vi "Begin.vi"(11 "Image Size":T1=enum."160x120") -> (0 "error out":errorcluster)   [LabVIEW 2011]
doc: "Called before other user functions, this VI is expected to open initial I/O refnums, load in file data, and do all program initialization. Notice that the <B>error out</B> terminal is simply used for data flow. Wiring it to other structures or subVIs ensures that this VI runs first."
uses:
  <vilib>/Rock Robotics/WPI/Camera/WPI_CameraImageSize.ctl
  <vilib>/Rock Robotics/SystemInterfaces/DIO/FPGA_DIOPWMChannel.ctl
  <vilib>/Rock Robotics/WPI/Joystick/WPI_JoystickDeviceEnum.ctl
  <vilib>/Rock Robotics/WPI/Camera/WPI_CameraWhite Balance Values.ctl
  <vilib>/Rock Robotics/WPI/Camera/WPI_CameraExposure Values.ctl
  <vilib>/Rock Robotics/WPI/Camera/WPI_CameraFrameRate.ctl
  <vilib>/Rock Robotics/SystemInterfaces/DIO/FPGA_DIOChannel.ctl
  <vilib>/Rock Robotics/SystemInterfaces/Typedef/FPGA_TypedefDigitalModule.ctl
  <vilib>/Rock Robotics/SystemInterfaces/Typedef/FPGA_TypedefSolenoidModule.ctl
  <vilib>/Rock Robotics/WPI/Solenoid/WPI_SolenoidChannel.ctl
  <vilib>/Rock Robotics/WPI/Encoder/WPI_EncoderType.ctl
  <vilib>/Rock Robotics/SystemInterfaces/DIO/FPGA_DIORelayChannel.ctl
  <vilib>/Rock Robotics/SystemInterfaces/AI/FPGA_AIGyroChannel.ctl
  <vilib>/Rock Robotics/SystemInterfaces/Typedef/FPGA_TypedefAnalogModuleForGyro.ctl
  <vilib>/Rock Robotics/WPI/Solenoid/WPI_SolenoidOpenSingle.vi
  <vilib>/Rock Robotics/WPI/Counter/WPI_CounterDigitalInputToDigitalSource.vi
  <vilib>/Rock Robotics/WPI/RobotDrive/WPI_RobotDriveOpen2MotorWithJaguar.vi
  <vilib>/Rock Robotics/WPI/RobotDrive/WPI_RobotDriveOpen4MotorWithJaguar.vi
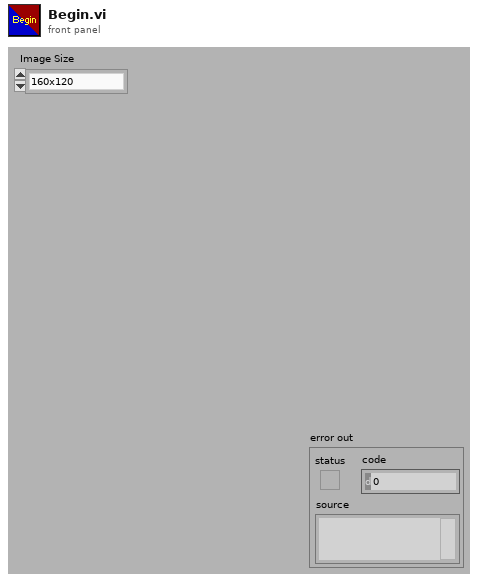
[diagram p1: front panel]
types:
  T1 = typedef "WPI_CameraImageSize.ctl" = enum16{"640x480", "320x240", "160x120"}
  T2 = typedef "FPGA_DIOChannel.ctl" = enum8{"DIO 1", "DIO 2", "DIO 3", "DIO 4", "DIO 5", "DIO 6", "DIO 7", "DIO 8", "DIO 9", "DIO 10", "DIO 11", "DIO 12", "DIO 13", "DIO 14", "Invalid"}
  T3 = typedef "FPGA_TypedefDigitalModule.ctl" = enum16{"Digital Module 1", "Digital Module 2"}
  T4 = typedef "WPI_EncoderType.ctl" = enum16{"1x", "2x", "4x"}
  T5 = typedef "FPGA_TypedefSolenoidModule.ctl" = enum16{"Solenoid Module 1", "Solenoid Module 2"}
  T6 = typedef "WPI_SolenoidChannel.ctl" = enum8{"Solenoid 1", "Solenoid 2", "Solenoid 3", "Solenoid 4", "Solenoid 5", "Solenoid 6", "Solenoid 7", "Solenoid 8", "Invalid"}
  T7 = typedef "FPGA_TypedefAnalogModuleForGyro.ctl" = enum16{"Analog Module 1"}
  T8 = typedef "FPGA_AIGyroChannel.ctl" = enum8{"AI 1", "AI 2", "Invalid"}
  T9 = typedef "FPGA_DIORelayChannel.ctl" = enum8{"Relay 1", "Relay 2", "Relay 3", "Relay 4", "Relay 5", "Relay 6", "Relay 7", "Relay 8", "Invalid"}
  T10 = typedef "FPGA_DIOPWMChannel.ctl" = enum8{"PWM 1", "PWM 2", "PWM 3", "PWM 4", "PWM 5", "PWM 6", "PWM 7", "PWM 8", "PWM 9", "PWM 10", "Invalid"}
  T11 = typedef "WPI_JoystickDeviceEnum.ctl" = enum16{"USB 1", "USB 2", "USB 3", "USB 4", "Kinect 1", "Kinect 2"}
  T12 = typedef "WPI_CameraFrameRate.ctl" = u32
  T13 = typedef "WPI_CameraExposure Values.ctl" = enum16{"Auto", "Flicker-free 50 Hz", "Flicker-free 60 Hz", "Hold current"}
  T14 = typedef "WPI_CameraWhite Balance Values.ctl" = enum16{"Auto", "Fixed indoor", "Fixed outdoor 1", "Fixed outdoor 2", "Fixed fluorescent 1", "Fixed fluorescent 2", "Hold current"}
  T15 = typedef "WPI_CompressorDevRef.ctl" = cluster{"DevStatus":errorcluster, "TaskVI":refnum<vi>, "Enabled":bool, "FIFO_enabled":refnum<k33>, "FIFO_relay":refnum<k33>}
  T16 = typedef "WPI_SolenoidDevRef.ctl" = cluster{"DevStatus":errorcluster, "Solenoid Module":T5, "Forward Solenoid Channel":T6, "Reverse Solenoid Channel":T6}
  T17 = typedef "WPI_DigitalInputDevRef.ctl" = cluster{"DevStatus":errorcluster, "DIO Channel":T2, "Digital Module":T3}
  T18 = typedef "WPI_JoystickDevRef.ctl" = cluster{"Device":T11}
  T19 = typedef "WPI_CameraDevRef.ctl" = cluster{"Camera Address":string, "CameraStatus":errorcluster, "Session ID":T20}
  T20 = typedef "WPI_CameraSessionID.ctl" = i32
  T21 = typedef "WPI_ServoDeviceRef.ctl" = cluster{"DeviceStatus":errorcluster, "Digital Module":T3, "PWM Channel":T10, "DeadBand":T22}
  T22 = typedef "WPI_PWMDeadband.ctl" = cluster{"Name":string, "maxPositivePwm":i32, "minPositivePwm":i32, "centerPwm":i32, "maxNegativePwm":i32, "minNegativePwm":i32, "angularRange":u16}
  T23 = typedef "WPI_RobotDriveDevRef.ctl" = cluster{"DevStatus":errorcluster, "Motors[]":T24[], "Square Inputs":bool, "Max Output":dbl}
  T24 = typedef "WPI_MotorControlDeviceRef.ctl" = cluster{"DeviceStatus":errorcluster, "Type":enum16{"PWM", "CAN"}, "PWM":cluster{"Digital Module":T3, "PWM Channel":T10, "DeadBand":T22}, "CAN":cluster{"Device Number":u8, "Control Mode":T25, "Semaphore":T26, "Max Vout":dbl}, "Invert":bool, "TransformRef":T27, "InvTransformRef":T27}
  T25 = typedef "WPI_CANJaguar_ControlMode.ctl" = enum8{"Percent VBus", "Current", "Speed", "Position", "Voltage"}
  T26 = typedef "Semaphore RefNum" = refnum<k1>
  T27 = typedef "WPI_PWMTransform_ConPane.ctl" = refnum<vi>
  T28 = typedef "FPGA_CounterEncoderSourceConvertionLVSourceType.ctl" = cluster{"DevStatus":errorcluster, "AnalogTriggerMode?":bool, "DigitalMode":cluster{"Digital Module":T3, "DIO Channel":T29}, "AnalogTriggerMode":cluster{"AnalogTriggerIndex":T30, "OutputType":T31}}
  T29 = typedef "FPGA_DIODigitalSourceChannel.ctl" = enum8{"DIO 1", "DIO 2", "DIO 3", "DIO 4", "DIO 5", "DIO 6", "DIO 7", "DIO 8", "DIO 9", "DIO 10", "DIO 11", "DIO 12", "DIO 13", "DIO 14", "Disabled"}
  T30 = typedef "FPGA_AnalogTriggerIndex.ctl" = enum8{"Trig 0", "Trig 1", "Trig 2", "Trig 3", "Trig 4", "Trig 5", "Trig 6", "Trig 7", "Invalid"}
  T31 = typedef "FPGA_AnalogTriggerOutType.ctl" = enum16{"InWindow", "TriggerState", "Rising", "Falling"}
  T32 = typedef "WPI_EncoderDevRef.ctl" = cluster{"DevStatus":errorcluster, "EncoderIndex":T33, "CounterIndex":T34, "DistancePerCount":dbl, "Decoding Type":T4}
  T33 = typedef "FPGA_EncoderIdx.ctl" = enum8{"Enc 0", "Enc 1", "Enc 2", "Enc 3", "Invalid"}
  T34 = typedef "FPGA_CounterCtrSystemIndex.ctl" = enum8{"Ctr 0", "Ctr 1", "Ctr 2", "Ctr 3", "Ctr 4", "Ctr 5", "Ctr 6", "Ctr 7", "Invalid"}
  T35 = typedef "WPI_GyroDevRef.ctl" = cluster{"DevStatus":errorcluster, "Analog Module":T36, "Analog Channel":T37, "Offset":dbl, "Gain (VoltsPerDegree/Second)":dbl}
  T36 = typedef "FPGA_TypedefAnalogModule.ctl" = enum16{"Analog Module 1", "Analog Module 2"}
  T37 = typedef "FPGA_AIChannel.ctl" = enum8{"AI 1", "AI 2", "AI 3", "AI 4", "AI 5", "AI 6", "AI 7", "AI 8", "Invalid"}
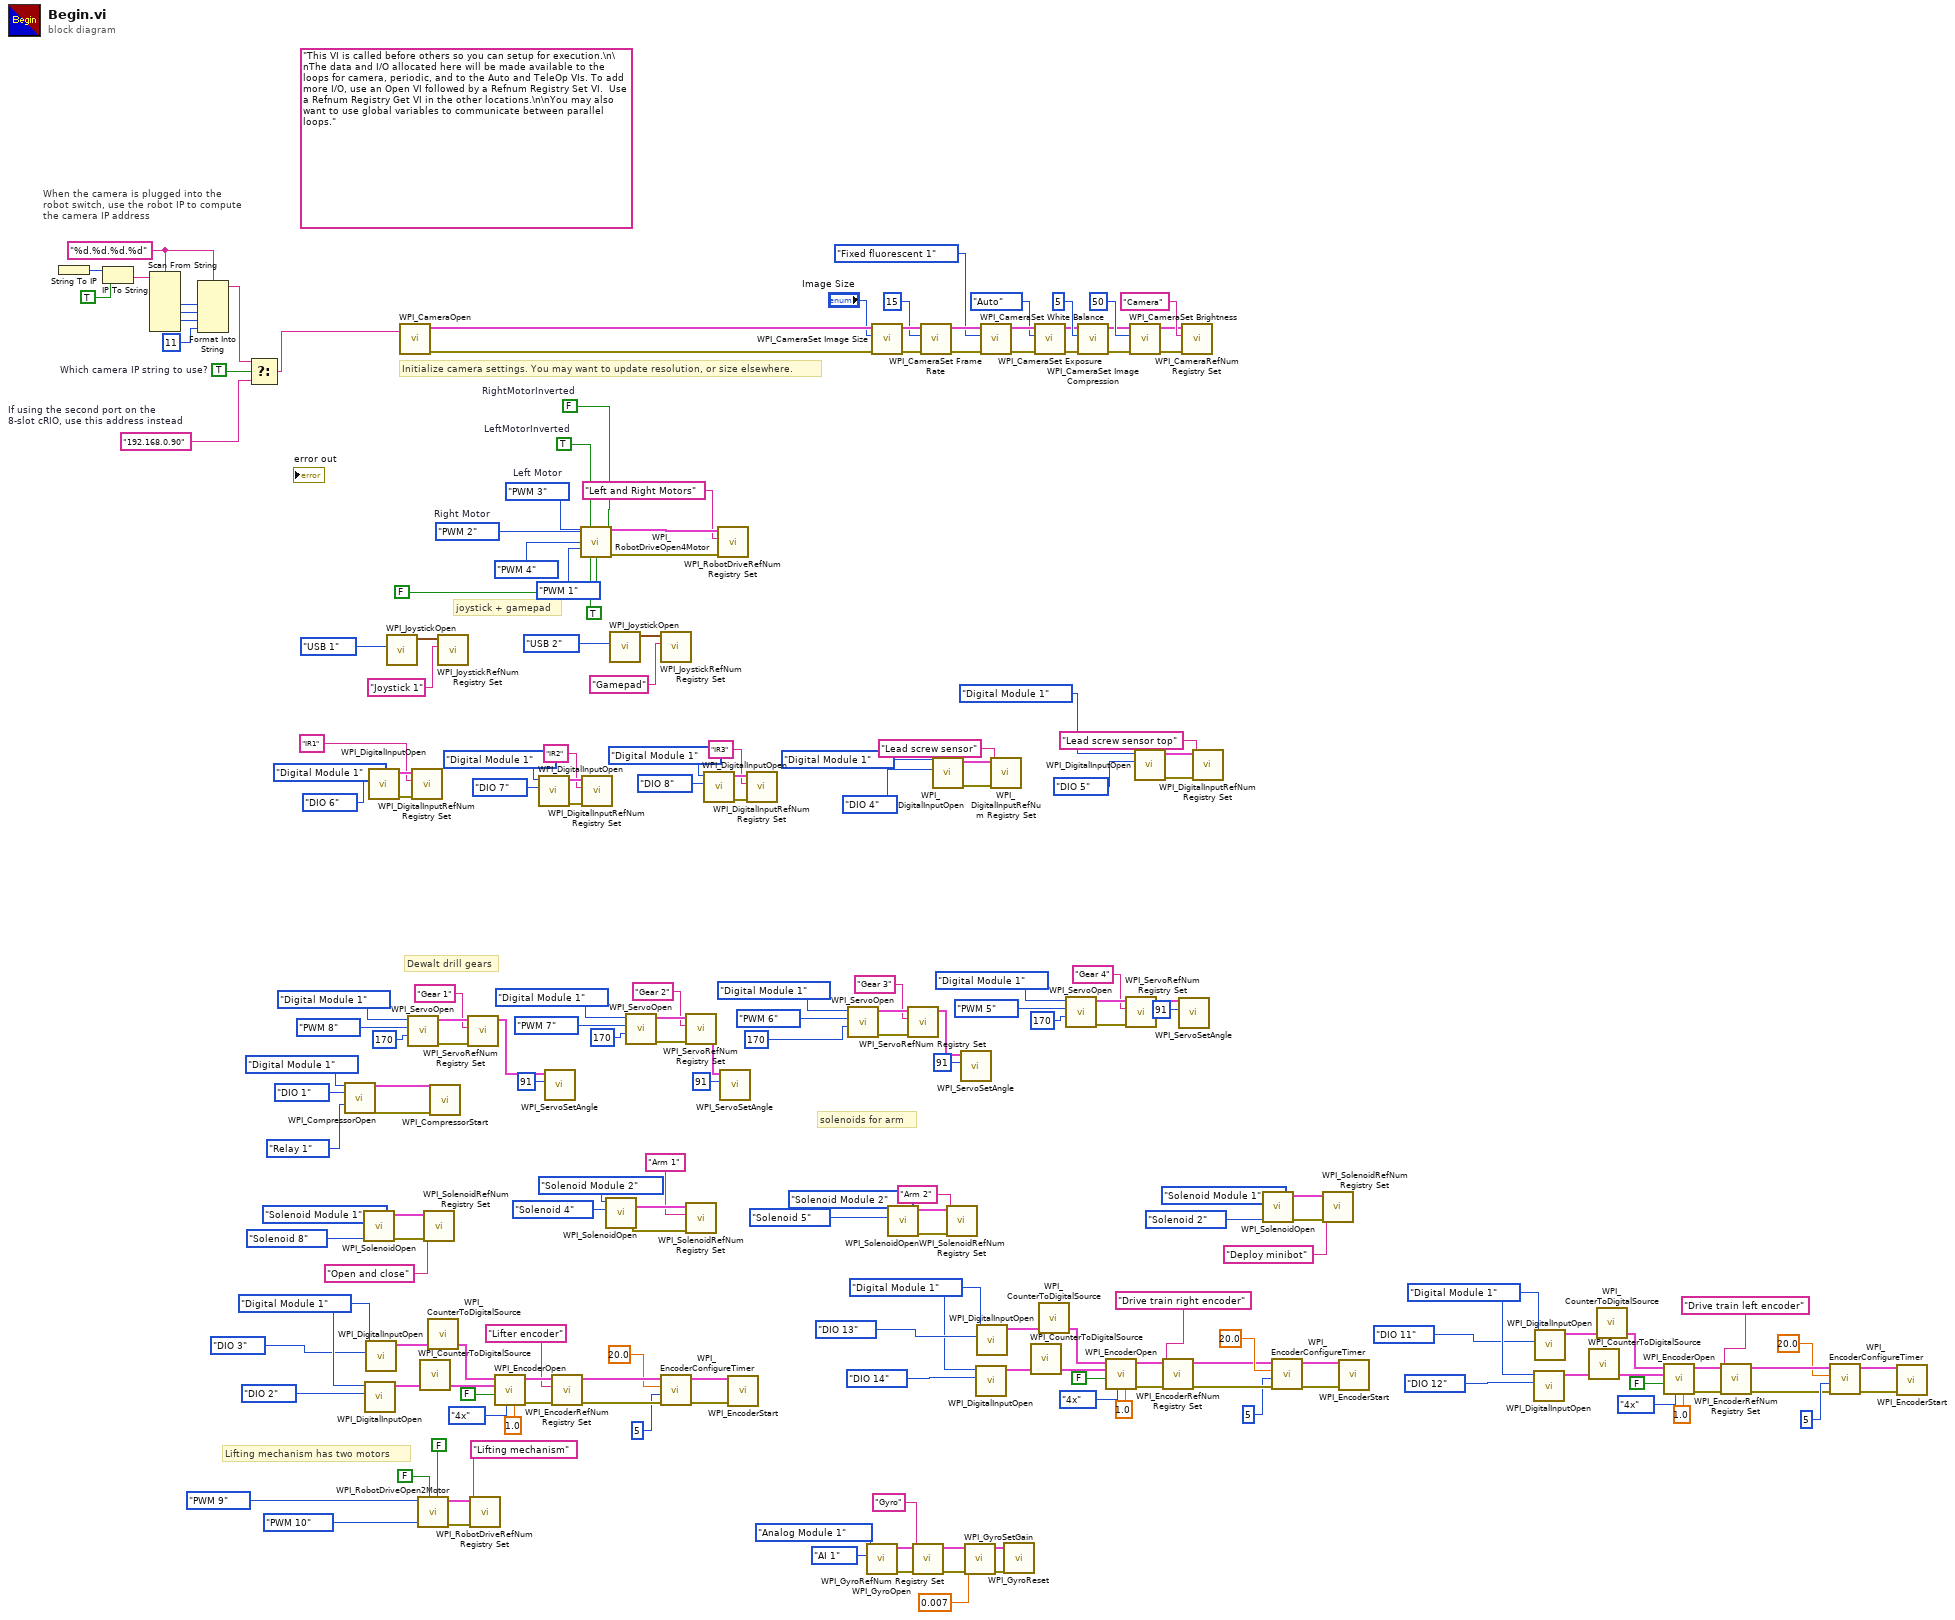
[diagram p0: block diagram]
diagram:
  w2 = TRUE  # Which camera IP string to use?
  w5 = "%d.%d.%d.%d" ("format string")
  w3 = "192.168.0.90"  # If using the second port on the 8-slot cRIO, use this address instead
  w33 = FPGA_TypedefDigitalModule."Digital Module 1" ("DIO Module (Slot 4)")
  w68 = FPGA_TypedefDigitalModule."Digital Module 1" ("DIO Module (Slot 4)")
  w106 = FPGA_TypedefDigitalModule."Digital Module 1" ("DIO Module (Slot 4)")
  (unwired) "This VI is called before others so you can setup for execution.\n\nThe data and I/O allocated here will be made available to the loops for camera, periodic, and to the Auto and TeleOp VIs. To add more I/O, use an Open VI followed by a Refnum Registry Set VI.  Use a Refnum Registry Get VI in the other locations.\n\nYou may also want to use global variables to communicate between parallel loops."
  w122 = FPGA_DIOPWMChannel."PWM 2"  # Right Motor
  w181 = FPGA_DIOPWMChannel."PWM 3"  # Left Motor
  w205 = TRUE  # LeftMotorInverted
  w206 = FALSE  # RightMotorInverted
  # "When the camera is plugged into the\nrobot switch, use the robot IP to compute\nthe camera IP address"
  # "Lifting mechanism has two motors"
  # "joystick + gamepad"
  # "Dewalt drill gears"
  # "solenoids for arm"
  # "Initialize camera settings. You may want to update resolution, or size elsewhere."
  n1 = String To IP() -> (0:w12:u32)  [unwired: 1 in]
  n2 = IP To String(1:TRUE ("dot notation? (F)"), 2:w12) -> (0:w10:string)
  n3 = Scan From String(format string=w5, input string=w10) -> (output 1=w9:i32, output 2=w8:i32, output 3=w7:i32)  [unwired: 7 in, 3 out]
  n4 = Format Into String(format string=w5, w9, w8, w7, 11 ("Compression")) -> (resulting string=w4:string)  [unwired: 2 in, 1 out]
  n5 = Select(t=w4, s=w2, f=w3) -> (s? t:f=w1:string)
  n6 = call <vilib>:"WPI_CompressorOpen.vi"("Pressure Switch Digital Module (Module 1)"=FPGA_TypedefDigitalModule."Digital Module 1" ("Pressure Switch DIO Module"), "Pressure Switch DIO Channel"=FPGA_DIOChannel."DIO 1", "Relay Channel"=FPGA_DIORelayChannel."Relay 1") -> ("CompressorDevRef"=w88:T15, "error out"=w87:errorcluster)  [unwired: 2 in, 9 out]
  n7 = call-poly <vilib>:"WPI_SolenoidOpen.vi"("Solenoid Channel"=WPI_SolenoidChannel."Solenoid 8", "Solenoid Module (Module 1)"=FPGA_TypedefSolenoidModule."Solenoid Module 1" ("Solenoid Module")) -> ("error out"=w133:errorcluster, "SolenoidDevRef"=w132:T16)  [unwired: 2 in, 6 out]
  n8 = call <vilib>:"WPI_DigitalInputOpen.vi"("DIO Channel"=FPGA_DIOChannel."DIO 2", "Digital Module (Module 1)"=w106) -> ("DigitalInputDevRef"=w108:T17)  [unwired: 1 in, 8 out]
  n9 = call <vilib>:"WPI_DigitalInputOpen.vi"("DIO Channel"=FPGA_DIOChannel."DIO 3", "Digital Module (Module 1)"=w106) -> ("DigitalInputDevRef"=w110:T17)  [unwired: 1 in, 8 out]
  n10 = call <vilib>:"WPI_DigitalInputOpen.vi"("DIO Channel"=FPGA_DIOChannel."DIO 6", "Digital Module (Module 1)"=FPGA_TypedefDigitalModule."Digital Module 1" ("DIO Module (Slot 4)")) -> ("error out"=w170:errorcluster, "DigitalInputDevRef"=w169:T17)  [unwired: 1 in, 7 out]
  n11 = call <vilib>:"WPI_JoystickOpen.vi"("JoystickDevice"=WPI_JoystickDeviceEnum."USB 1") -> ("JoystickDevRef"=w201:T18)  [unwired: 10 out]
  n12 = call <vilib>:"WPI_CameraOpen.vi"("Camera Address"=w1) -> ("error out"=w190:errorcluster, "CameraDevRef"=w191:T19)  [unwired: 1 in, 8 out]
  n13 = call <vilib>:"WPI_ServoOpen.vi"("Angular Range"=u16 170, "PWM Channel"=FPGA_DIOPWMChannel."PWM 8", "Digital Module (Module 1)"=FPGA_TypedefDigitalModule."Digital Module 1" ("DIO Module (Slot 4)")) -> ("error out"=w144:errorcluster, "ServoDeviceRef"=w145:T21)  [unwired: 1 in, 6 out]
  n14 = call <vilib>:"WPI_DigitalInputRefNum Registry Set.vi"("error in (no error)"=w170, "refnum name"="IR1", "DigitalInputDevRef"=w169) -> ()  [unwired: 9 out]
  n15 = call-poly <vilib>:"WPI_RobotDriveOpen2Motor.vi"("Right Motor Inverted"=FALSE, "Left Motor Inverted"=FALSE, "Right Motor"=FPGA_DIOPWMChannel."PWM 10" ("PWM Channel"), "Left Motor"=FPGA_DIOPWMChannel."PWM 9") -> ("error out"=w121:errorcluster, "RobotDriveDevRef"=w102:T23)  [unwired: 1 in, 5 out]
  n16 = call-poly <vilib>:"WPI_CounterToDigitalSource.vi"("DigitalInputDevRef"=w108) -> ("Digital Source"=w107:T28)  [unwired: 6 out]
  n17 = call <vilib>:"WPI_SolenoidRefNum Registry Set.vi"("error in (no error)"=w133, "refnum name"="Open and close", "SolenoidDevRef"=w132) -> ()  [unwired: 9 out]
  n18 = call-poly <vilib>:"WPI_CounterToDigitalSource.vi"("DigitalInputDevRef"=w110) -> ("Digital Source"=w109:T28)  [unwired: 6 out]
  n19 = call <vilib>:"WPI_CompressorStart.vi"("error in (no error)"=w87, "CompressorDevRef"=w88) -> ()  [unwired: 10 out]
  n20 = call <vilib>:"WPI_JoystickRefNum Registry Set.vi"("refnum name"="Joystick 1", "JoystickDevRef"=w201) -> ()  [unwired: 1 in, 9 out]
  n21 = call <vilib>:"WPI_ServoRefNum Registry Set.vi"("error in (no error)"=w144, "refnum name"="Gear 1", "ServoDeviceRef"=w145) -> ("ServoDeviceRef"=w20:T21)  [unwired: 8 out]
  n22 = call <vilib>:"WPI_RobotDriveRefNum Registry Set.vi"("error in (no error)"=w121, "refnum name"="Lifting mechanism", "RobotDriveDevRef"=w102) -> ()  [unwired: 9 out]
  n23 = call <vilib>:"WPI_EncoderOpen.vi"("DistancePerCount"=1.0, "Decoding Type"=WPI_EncoderType."4x", "Invert Direction (False)"=FALSE, "BSource"=w107, "ASource"=w109) -> ("error out"=w118:errorcluster, "EncoderDevRef"=w117:T32)  [unwired: 3 in, 2 out]
  n24 = call <vilib>:"WPI_DigitalInputOpen.vi"("DIO Channel"=FPGA_DIOChannel."DIO 7", "Digital Module (Module 1)"=FPGA_TypedefDigitalModule."Digital Module 1" ("DIO Module (Slot 4)")) -> ("error out"=w168:errorcluster, "DigitalInputDevRef"=w167:T17)  [unwired: 1 in, 7 out]
  n25 = call <vilib>:"WPI_ServoSetAngle.vi"("Angle"=91, "ServoDeviceRef"=w20) -> ()  [unwired: 1 in, 9 out]
  n26 = call <vilib>:"WPI_EncoderRefNum Registry Set.vi"("error in (no error)"=w118, "refnum name"="Lifter encoder", "EncoderDevRef"=w117) -> ("error out"=w83:errorcluster, "EncoderDevRef"=w84:T32)  [unwired: 7 out]
  n27 = call-poly <vilib>:"WPI_RobotDriveOpen4Motor.vi"("Rear Left Motor"=w181, "Rear Left Motor Inverted"=w205, "Rear Right Motor Inverted"=w206, "Rear Right Motor"=w122, "Front Left Motor"=FPGA_DIOPWMChannel."PWM 4", "Front Right Motor"=FPGA_DIOPWMChannel."PWM 1", "Front Left Motor Inverted"=TRUE, "Front Right Motor Inverted"=FALSE) -> ("RobotDriveDevRef"=w203:T23, "error out"=w199:errorcluster)  [unwired: 1 in, 5 out]
  n28 = call <vilib>:"WPI_DigitalInputRefNum Registry Set.vi"("error in (no error)"=w168, "refnum name"="IR2", "DigitalInputDevRef"=w167) -> ()  [unwired: 9 out]
  n29 = call-poly <vilib>:"WPI_SolenoidOpen.vi"("Solenoid Channel"=WPI_SolenoidChannel."Solenoid 4", "Solenoid Module (Module 1)"=FPGA_TypedefSolenoidModule."Solenoid Module 2" ("Solenoid Module")) -> ("error out"=w131:errorcluster, "SolenoidDevRef"=w130:T16)  [unwired: 2 in, 6 out]
  n30 = call <vilib>:"WPI_JoystickOpen.vi"("JoystickDevice"=WPI_JoystickDeviceEnum."USB 2") -> ("JoystickDevRef"=w124:T18)  [unwired: 10 out]
  n31 = call <vilib>:"WPI_ServoOpen.vi"("Angular Range"=u16 170, "PWM Channel"=FPGA_DIOPWMChannel."PWM 7", "Digital Module (Module 1)"=FPGA_TypedefDigitalModule."Digital Module 1" ("DIO Module (Slot 4)")) -> ("error out"=w146:errorcluster, "ServoDeviceRef"=w149:T21)  [unwired: 1 in, 6 out]
  n32 = call <vilib>:"WPI_JoystickRefNum Registry Set.vi"("refnum name"="Gamepad", "JoystickDevRef"=w124) -> ()  [unwired: 1 in, 9 out]
  n33 = call <vilib>:"WPI_EncoderConfigureTimer.vi"("error in (no error)"=w83, "Number Samples to Average"=u8 5, "Minimum Rate"=20.0, "EncoderDevRef"=w84) -> ("error out"=w79:errorcluster, "EncoderDevRef"=w80:T32)  [unwired: 6 out]
  n34 = call <vilib>:"WPI_ServoRefNum Registry Set.vi"("error in (no error)"=w146, "refnum name"="Gear 2", "ServoDeviceRef"=w149) -> ("ServoDeviceRef"=w18:T21)  [unwired: 8 out]
  n35 = call <vilib>:"WPI_SolenoidRefNum Registry Set.vi"("error in (no error)"=w131, "refnum name"="Arm 1", "SolenoidDevRef"=w130) -> ()  [unwired: 9 out]
  n36 = call <vilib>:"WPI_DigitalInputOpen.vi"("DIO Channel"=FPGA_DIOChannel."DIO 8", "Digital Module (Module 1)"=FPGA_TypedefDigitalModule."Digital Module 1" ("DIO Module (Slot 4)")) -> ("error out"=w166:errorcluster, "DigitalInputDevRef"=w165:T17)  [unwired: 1 in, 7 out]
  n37 = call <vilib>:"WPI_RobotDriveRefNum Registry Set.vi"("error in (no error)"=w199, "refnum name"="Left and Right Motors", "RobotDriveDevRef"=w203) -> ()  [unwired: 9 out]
  n38 = call <vilib>:"WPI_ServoSetAngle.vi"("Angle"=91, "ServoDeviceRef"=w18) -> ()  [unwired: 1 in, 9 out]
  n39 = call <vilib>:"WPI_EncoderStart.vi"("error in (no error)"=w79, "EncoderDevRef"=w80) -> ()  [unwired: 10 out]
  n40 = call <vilib>:"WPI_DigitalInputRefNum Registry Set.vi"("error in (no error)"=w166, "refnum name"="IR3", "DigitalInputDevRef"=w165) -> ()  [unwired: 9 out]
  n41 = call <vilib>:"WPI_ServoOpen.vi"("Angular Range"=u16 170, "PWM Channel"=FPGA_DIOPWMChannel."PWM 6", "Digital Module (Module 1)"=FPGA_TypedefDigitalModule."Digital Module 1" ("DIO Module (Slot 4)")) -> ("error out"=w148:errorcluster, "ServoDeviceRef"=w147:T21)  [unwired: 1 in, 6 out]
  n42 = call <vilib>:"WPI_GyroOpen.vi"("Analog Channel"=FPGA_AIGyroChannel."AI 1", "Analog Module (Module 1)"=FPGA_TypedefAnalogModuleForGyro."Analog Module 1" ("Analog Module (Slot 1)")) -> ("error out"=w57:errorcluster, "GyroDevRef"=w56:T35)  [unwired: 4 in, 4 out]
  n43 = call <vilib>:"WPI_CameraSet Image Size.vi"("error in (no error)"=w190, "Image Size"="Image Size", "CameraDevRef"=w191) -> ("error out"=w189:errorcluster, "CameraDevRef Out"=w192:T19)  [unwired: 7 out]
  n44 = call-poly <vilib>:"WPI_SolenoidOpen.vi"("Solenoid Channel"=WPI_SolenoidChannel."Solenoid 5", "Solenoid Module (Module 1)"=FPGA_TypedefSolenoidModule."Solenoid Module 2" ("Solenoid Module")) -> ("error out"=w47:errorcluster, "SolenoidDevRef"=w46:T16)  [unwired: 2 in, 6 out]
  n45 = call <vilib>:"WPI_ServoRefNum Registry Set.vi"("error in (no error)"=w148, "refnum name"="Gear 3", "ServoDeviceRef"=w147) -> ("ServoDeviceRef"=w16:T21)  [unwired: 8 out]
  n46 = call <vilib>:"WPI_GyroRefNum Registry Set.vi"("error in (no error)"=w57, "refnum name"="Gyro", "GyroDevRef"=w56) -> ("error out"=w44:errorcluster, "GyroDevRef"=w43:T35)  [unwired: 7 out]
  n47 = call <vilib>:"WPI_CameraSet Frame Rate.vi"("error in (no error)"=w189, "Frame Rate (fps)"=T12 15, "CameraDevRef"=w192) -> ("error out"=w188:errorcluster, "CameraDevRef Out"=w194:T19)  [unwired: 7 out]
  n48 = call <vilib>:"WPI_DigitalInputOpen.vi"("DIO Channel"=FPGA_DIOChannel."DIO 4", "Digital Module (Module 1)"=FPGA_TypedefDigitalModule."Digital Module 1" ("DIO Module (Slot 4)")) -> ("error out"=w115:errorcluster, "DigitalInputDevRef"=w114:T17)  [unwired: 1 in, 7 out]
  n49 = call <vilib>:"WPI_SolenoidRefNum Registry Set.vi"("error in (no error)"=w47, "refnum name"="Arm 2", "SolenoidDevRef"=w46) -> ()  [unwired: 9 out]
  n50 = call <vilib>:"WPI_ServoSetAngle.vi"("Angle"=91, "ServoDeviceRef"=w16) -> ()  [unwired: 1 in, 9 out]
  n51 = call <vilib>:"WPI_GyroSetGain.vi"("error in (no error)"=w44, "Gain (VoltsPerDegree/Second)"=0.007, "GyroDevRef"=w43) -> ("error out"=w22:errorcluster, "GyroDevRef"=w21:T35)  [unwired: 7 out]
  n52 = call <vilib>:"WPI_DigitalInputOpen.vi"("DIO Channel"=FPGA_DIOChannel."DIO 14", "Digital Module (Module 1)"=w68) -> ("DigitalInputDevRef"=w66:T17)  [unwired: 1 in, 8 out]
  n53 = call <vilib>:"WPI_DigitalInputOpen.vi"("DIO Channel"=FPGA_DIOChannel."DIO 13", "Digital Module (Module 1)"=w68) -> ("DigitalInputDevRef"=w64:T17)  [unwired: 1 in, 8 out]
  n54 = call <vilib>:"WPI_CameraSet White Balance.vi"("error in (no error)"=w188, "White Balance"=WPI_CameraWhite_Balance_Values."Fixed fluorescent 1", "CameraDevRef"=w194) -> ("error out"=w187:errorcluster, "CameraDevRef Out"=w193:T19)  [unwired: 7 out]
  n55 = call <vilib>:"WPI_DigitalInputRefNum Registry Set.vi"("error in (no error)"=w115, "refnum name"="Lead screw sensor", "DigitalInputDevRef"=w114) -> ()  [unwired: 9 out]
  n56 = call <vilib>:"WPI_GyroReset.vi"("error in (no error)"=w22, "GyroDevRef"=w21) -> ()  [unwired: 10 out]
  n57 = call-poly <vilib>:"WPI_CounterToDigitalSource.vi"("DigitalInputDevRef"=w66) -> ("Digital Source"=w67:T28)  [unwired: 6 out]
  n58 = call <vilib>:"WPI_CameraSet Exposure.vi"("error in (no error)"=w187, "Exposure"=WPI_CameraExposure_Values."Auto", "CameraDevRef"=w193) -> ("error out"=w186:errorcluster, "CameraDevRef Out"=w196:T19)  [unwired: 7 out]
  n59 = call-poly <vilib>:"WPI_CounterToDigitalSource.vi"("DigitalInputDevRef"=w64) -> ("Digital Source"=w65:T28)  [unwired: 6 out]
  n60 = call <vilib>:"WPI_ServoOpen.vi"("Angular Range"=u16 170, "PWM Channel"=FPGA_DIOPWMChannel."PWM 5", "Digital Module (Module 1)"=FPGA_TypedefDigitalModule."Digital Module 1" ("DIO Module (Slot 4)")) -> ("error out"=w143:errorcluster, "ServoDeviceRef"=w142:T21)  [unwired: 1 in, 6 out]
  n61 = call <vilib>:"WPI_CameraSet Image Compression.vi"("error in (no error)"=w186, "Compression"=5, "CameraDevRef"=w196) -> ("error out"=w185:errorcluster, "CameraDevRef Out"=w195:T19)  [unwired: 7 out]
  n62 = call <vilib>:"WPI_EncoderOpen.vi"("DistancePerCount"=1.0, "Decoding Type"=WPI_EncoderType."4x", "Invert Direction (False)"=FALSE, "BSource"=w67, "ASource"=w65) -> ("error out"=w61:errorcluster, "EncoderDevRef"=w62:T32)  [unwired: 3 in, 2 out]
  n63 = call <vilib>:"WPI_ServoRefNum Registry Set.vi"("error in (no error)"=w143, "refnum name"="Gear 4", "ServoDeviceRef"=w142) -> ("ServoDeviceRef"=w14:T21)  [unwired: 8 out]
  n64 = call <vilib>:"WPI_CameraSet Brightness.vi"("error in (no error)"=w185, "Brightness"=50, "CameraDevRef"=w195) -> ("error out"=w183:errorcluster, "CameraDevRef Out"=w184:T19)  [unwired: 7 out]
  n65 = call <vilib>:"WPI_DigitalInputOpen.vi"("DIO Channel"=FPGA_DIOChannel."DIO 5", "Digital Module (Module 1)"=FPGA_TypedefDigitalModule."Digital Module 1" ("DIO Module (Slot 4)")) -> ("error out"=w94:errorcluster, "DigitalInputDevRef"=w95:T17)  [unwired: 1 in, 7 out]
  n66 = call <vilib>:"WPI_EncoderRefNum Registry Set.vi"("error in (no error)"=w61, "refnum name"="Drive train right encoder", "EncoderDevRef"=w62) -> ("error out"=w75:errorcluster, "EncoderDevRef"=w74:T32)  [unwired: 7 out]
  n67 = call <vilib>:"WPI_ServoSetAngle.vi"("Angle"=91, "ServoDeviceRef"=w14) -> ()  [unwired: 1 in, 9 out]
  n68 = call <vilib>:"WPI_CameraRefNum Registry Set.vi"("error in (no error)"=w183, "refnum name"="Camera", "CameraDevRef"=w184) -> ()  [unwired: 9 out]
  n69 = call <vilib>:"WPI_DigitalInputRefNum Registry Set.vi"("error in (no error)"=w94, "refnum name"="Lead screw sensor top", "DigitalInputDevRef"=w95) -> ()  [unwired: 9 out]
  n70 = call-poly <vilib>:"WPI_SolenoidOpen.vi"("Solenoid Channel"=WPI_SolenoidChannel."Solenoid 2", "Solenoid Module (Module 1)"=FPGA_TypedefSolenoidModule."Solenoid Module 1" ("Solenoid Module")) -> ("error out"=w52:errorcluster, "SolenoidDevRef"=w53:T16)  [unwired: 2 in, 6 out]
  n71 = call <vilib>:"WPI_EncoderConfigureTimer.vi"("error in (no error)"=w75, "Number Samples to Average"=u8 5, "Minimum Rate"=20.0, "EncoderDevRef"=w74) -> ("error out"=w78:errorcluster, "EncoderDevRef"=w77:T32)  [unwired: 6 out]
  n72 = call <vilib>:"WPI_SolenoidRefNum Registry Set.vi"("error in (no error)"=w52, "refnum name"="Deploy minibot", "SolenoidDevRef"=w53) -> ()  [unwired: 9 out]
  n73 = call <vilib>:"WPI_EncoderStart.vi"("error in (no error)"=w78, "EncoderDevRef"=w77) -> ()  [unwired: 10 out]
  n74 = call <vilib>:"WPI_DigitalInputOpen.vi"("DIO Channel"=FPGA_DIOChannel."DIO 12", "Digital Module (Module 1)"=w33) -> ("DigitalInputDevRef"=w35:T17)  [unwired: 1 in, 8 out]
  n75 = call <vilib>:"WPI_DigitalInputOpen.vi"("DIO Channel"=FPGA_DIOChannel."DIO 11", "Digital Module (Module 1)"=w33) -> ("DigitalInputDevRef"=w37:T17)  [unwired: 1 in, 8 out]
  n76 = call-poly <vilib>:"WPI_CounterToDigitalSource.vi"("DigitalInputDevRef"=w35) -> ("Digital Source"=w34:T28)  [unwired: 6 out]
  n77 = call-poly <vilib>:"WPI_CounterToDigitalSource.vi"("DigitalInputDevRef"=w37) -> ("Digital Source"=w36:T28)  [unwired: 6 out]
  n78 = call <vilib>:"WPI_EncoderOpen.vi"("DistancePerCount"=1.0, "Decoding Type"=WPI_EncoderType."4x", "Invert Direction (False)"=FALSE, "BSource"=w34, "ASource"=w36) -> ("error out"=w40:errorcluster, "EncoderDevRef"=w39:T32)  [unwired: 3 in, 2 out]
  n79 = call <vilib>:"WPI_EncoderRefNum Registry Set.vi"("error in (no error)"=w40, "refnum name"="Drive train left encoder", "EncoderDevRef"=w39) -> ("error out"=w26:errorcluster, "EncoderDevRef"=w27:T32)  [unwired: 7 out]
  n80 = call <vilib>:"WPI_EncoderConfigureTimer.vi"("error in (no error)"=w26, "Number Samples to Average"=u8 5, "Minimum Rate"=20.0, "EncoderDevRef"=w27) -> ("error out"=w23:errorcluster, "EncoderDevRef"=w24:T32)  [unwired: 6 out]
  n81 = call <vilib>:"WPI_EncoderStart.vi"("error in (no error)"=w23, "EncoderDevRef"=w24) -> ()  [unwired: 10 out]
